vi "New Report.vi"(4 "error in (no error)":errorcluster, 6 "report type":enum16{"Standard Report", "HTML"}(ring)) -> (0 "error out":errorcluster, 3 "report out":T1)   [LabVIEW 2015]
doc: "Creates a new report."
uses:
  <vilib>/Utility/NIReport.llb/Generate Report Object Reference.ctl
  <vilib>/Utility/NIReport.llb/NI_report.lvclass
panel:
  in  "NIReports.Report":refnum<k7>
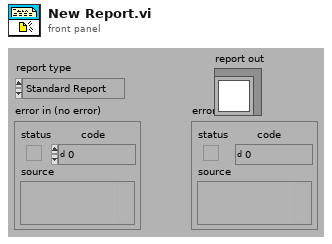
[diagram p1: front panel]
types:
  T1 = typedef "Generate Report Object Reference.ctl" = refnum<class "NI_report.lvclass">
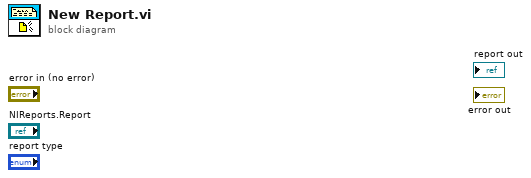
[diagram p0: block diagram]
diagram:
